vi "Cost.vi"(8 "error in (no error)":errorcluster, 11 "Espresso in":refnum<class "Espresso.lvclass">) -> (0 "error out":errorcluster, 2 "Cost":dbl, 3 "Espresso out":refnum<class "Espresso.lvclass">)   [LabVIEW 2020, in "Espresso.lvclass"]
uses:
  Espresso.lvclass
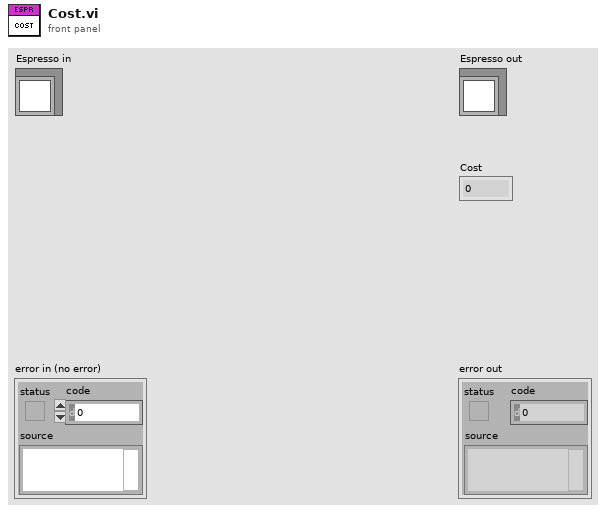
[diagram p1: front panel]
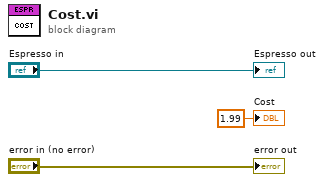
[diagram p0: block diagram]
diagram:
  "error out" <- "error in (no error)"
  "Espresso out" <- "Espresso in"
  "Cost" <- 1.99 ("Cost")
